vi "Read Switch.vi"(8 "error in (no error)":errorcluster, 11 "Z_HSw in":refnum<class "Z_OnSw.lvclass">) -> (0 "error out":errorcluster, 2 "Switch":bool, 3 "Z_HSw out":refnum<class "Z_OnSw.lvclass">)   [LabVIEW 2019, in "Z_OnSw.lvclass"]
uses:
  Z_OnSw.lvclass
  Z_OnSw.lvclass/Z_OnSw.ctl
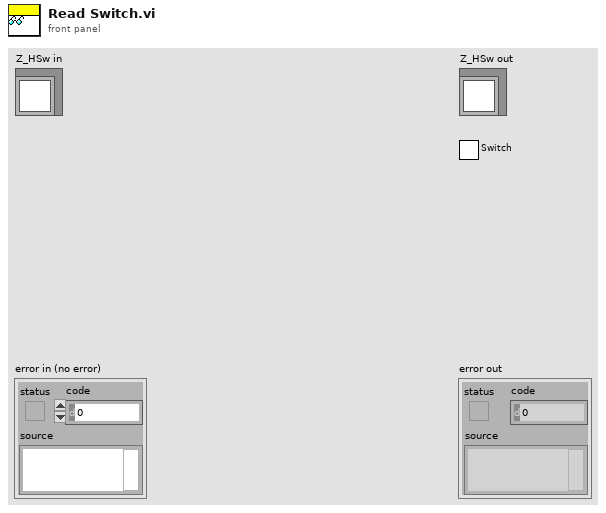
[diagram p1: front panel]
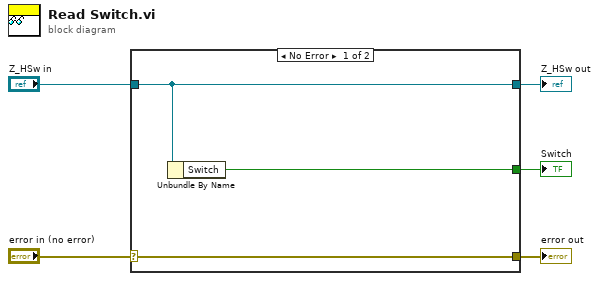
[diagram p0: block diagram]
diagram:
  n1 = case shown="No Error" "error in (no error)" {
    selector: "error in (no error)" -> [w8 w9]
    tunnel: [w8 w9] -> w4
    tunnel: [w7 w10] -> w2
    tunnel: "Z_HSw in" -> [w7 w10]
    tunnel: [w6 _] -> w1
    frame No Error {
      n2 = Unbundle By Name(w7) -> ("Switch"=w6:bool)
    }
    frame Error {
    }
  }
  "error out" <- w4
  "Z_HSw out" <- w2
  "Switch" <- w1
